vi "in_2d spline interpolants.vi"(10 "X row":dbl[](array[numeric]), 11 "Z matrix":dbl[][](array[numeric])) -> (3 "2d spline interpolants":dbl[][](array[numeric]) format="%_6g")   [LabVIEW 2017, in "NI_Gmath.lvlib"]
uses:
  <vilib>/gmath/NI_Gmath.lvlib
  <vilib>/Analysis/NI_AALPro.lvlib
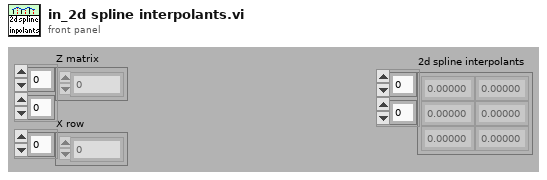
[diagram p1: front panel]
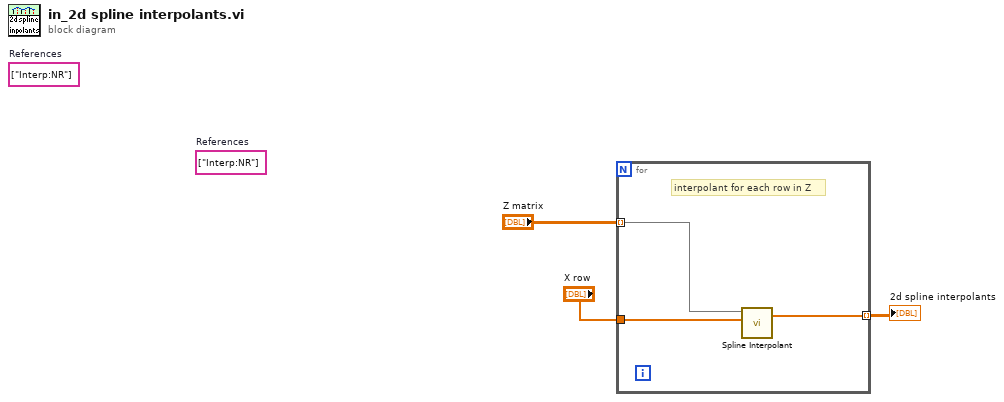
[diagram p0: block diagram]
diagram:
  (unwired) string[] ["Interp:NR"]  # References
  (unwired) string[] ["Interp:NR"]  # References
  n1 = for {
    tunnel: "Z matrix" -> [w6] mode=indexing
    tunnel: "X row" -> [w5]
    tunnel: [w4] -> w1 mode=indexing
    # "interpolant for each row in Z"
    n2 = call <vilib>:"Spline Interpolant.vi"("X"=w5, "Y"=w6) -> ("Interpolant"=w4:dbl[])  [unwired: 2 in, 1 out]
  }
  "2d spline interpolants" <- w1
